vi "Abort Motion.vi"(8 "error in (no error)":errorcluster, 11 "Fine SIM Motion Controller in":refnum<class "Fine SIM Motion Controller.lvclass">) -> (0 "error out":errorcluster, 3 "Fine SIM Motion Controller out":refnum<class "Fine SIM Motion Controller.lvclass">)   [LabVIEW 2022 SP3, in "Fine SIM Motion Controller.lvclass"]
uses:
  Fine SIM Motion Controller.lvclass
  Fine SIM Motion Controller.lvclass/Fine SIM Motion Controller.ctl
  Motion Controller/Homing Status.ctl
  Motion Controller/Parent SIM Motion Controller.lvclass
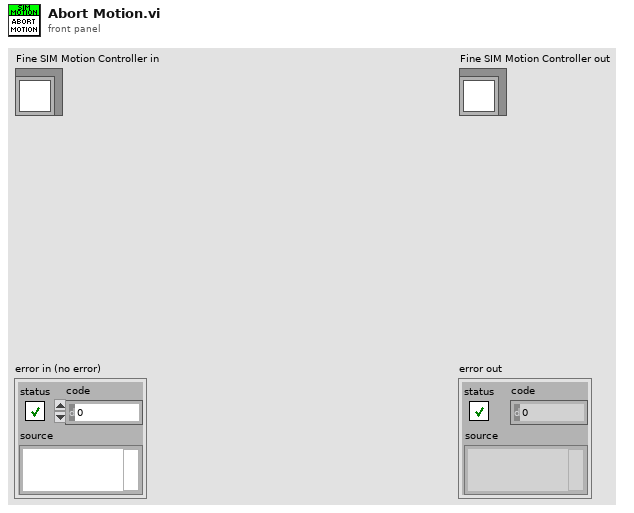
[diagram p1: front panel]
types:
  T1 = typedef "Parent SIM Motion Controller.lvclass/Homing Status.ctl" = enum16{"Idle", "Inital Home Motion", "Final Home Motion", "Done Homing"}
  T2 = typedef "Parent SIM Motion Controller.lvclass/Axis Data.ctl" = cluster{"Axis Parameters":T3, "Axis Settings":T4, "Time Stamp":timestamp}
  T3 = typedef "Parent SIM Motion Controller.lvclass/Axis Parameters.ctl" = cluster{"Moving":bool, "Homed":bool, "Desired Position":dbl, "Current Positon":dbl, "Current Speed":dbl, "Home Status":T1}
  T4 = typedef "Parent SIM Motion Controller.lvclass/Axis Settings.ctl" = cluster{"Speed":dbl, "Acceleration":dbl}
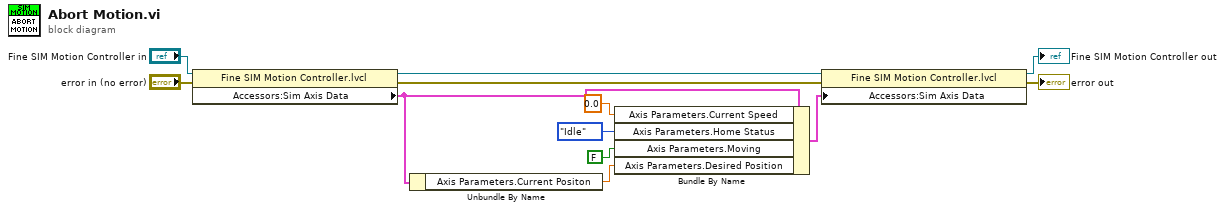
[diagram p0: block diagram]
diagram:
  n1 = property class="Fine SIM Motion Controller.lvcl"(reference="Fine SIM Motion Controller in", error in="error in (no error)") -> (reference out=w11:refnum<class "Fine SIM Motion Controller.lvclass">, error out=w2:errorcluster, "Accessors:Sim Axis Data"=w9:T2)
  n2 = Unbundle By Name(w9) -> ("Axis Parameters.Current Positon"=w5:dbl)
  n3 = Bundle By Name(cluster=w9, "Axis Parameters.Current Speed"=0.0, "Axis Parameters.Home Status"=Homing_Status."Idle", "Axis Parameters.Moving"=FALSE, "Axis Parameters.Desired Position"=w5) -> (w4:T2)
  n4 = property class="Fine SIM Motion Controller.lvcl"(reference=w11, error in=w2, "Accessors:Sim Axis Data"=w4) -> (reference out=→"Fine SIM Motion Controller out":refnum<class "Fine SIM Motion Controller.lvclass">, error out=→"error out":errorcluster)
